vi "Write Motor Port.vi"(10 "Motor Port":refnum<visa-resource-name>="COM4", 11 "Device Manager in":refnum<class "Device Manager.lvclass">) -> (3 "Device Manager out":refnum<class "Device Manager.lvclass">)   [LabVIEW 2020, in "Device Manager.lvlib" / "Device Manager.lvclass"]
uses:
  Device Manager.lvclass
  Device Manager.lvclass/Device Manager.ctl
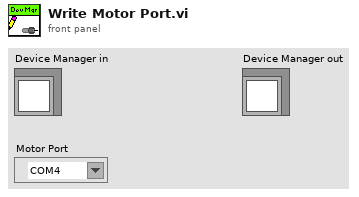
[diagram p1: front panel]
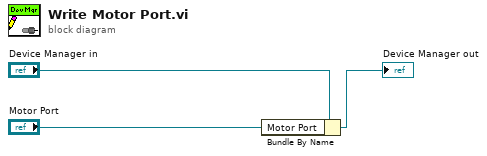
[diagram p0: block diagram]
diagram:
  n1 = Bundle By Name(cluster="Device Manager in", "Motor Port"="Motor Port") -> (→"Device Manager out":refnum<class "Device Manager.lvclass">)
